vi "Dig Test.vi"   [LabVIEW 2017, in "Tests.lvlib"]
uses:
  Tests.lvlib
  src/Toolkit VIs/Toolkit VIs.lvlib
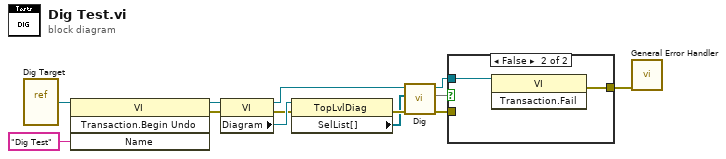
[diagram p0: block diagram]
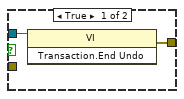
[diagram p2: hidden frame]
diagram:
  n1 = vi-ref "Dig Target.vi"() -> (w7:refnum<vi>)
  n2 = invoke class="VI" method="Transaction.Begin Undo"(reference=w7, "Name"="Dig Test") -> (reference out=w11:refnum<vi>, error out=w9:errorcluster)  [unwired: 2 in, 2 out]
  n3 = property class="VI"(reference=w11, error in=w9) -> (reference out=w6:refnum<vi>, error out=w12:errorcluster, "Diagram"=w13:refnum<vi>)
  n4 = property class="TopLvlDiag"(reference=w13, error in=w12) -> (error out=w8:errorcluster, "SelList[]"=w5:refnum<vi>[])  [unwired: 1 out]
  n5 = call "Dig.vi"("Error In"=w8, "Selection List[]"=w5, "VI In"=w6) -> ("Error Out"=w3:errorcluster, 2:w2, "VI Out"=w4:refnum<vi>)  [unwired: 6 in]
  n6 = case shown="False" w2 {
    tunnel: [w15 w17] -> w1
    tunnel: w4 -> [w14 w16]
    tunnel: w3 -> [_ _]
    frame True {
      n7 = invoke class="VI" method="Transaction.End Undo"(reference=w14) -> (error out=w15:errorcluster)  [unwired: 2 in, 2 out]
    }
    frame False {
      n8 = invoke class="VI" method="Transaction.Fail"(reference=w16) -> (error out=w17:errorcluster)  [unwired: 2 in, 2 out]
    }
  }
  n9 = call <vilib>:"General Error Handler.vi"("error in (no error)"=w1) -> ()  [unwired: 10 in, 5 out]
